vi "RT Image stream to FPGA.vi"() -> ()   [LabVIEW 2015]
uses:
  <vilib>/userdefined/High Color/IMAQdx.ctl
  <vilib>/vision/driver/IMAQdx.llb/IMAQdx Acquisition Mode.ctl
  <vilib>/vision/driver/IMAQdx.llb/IMAQdx Buffer Number Mode.ctl
  <vilib>/FPGAPlugInAG/cRIO-9030/niLvFpga_Open_cRIO-9030.vi
  <vilib>/rvi/interface/common/dynamic/niFpgaDynamicAddResources.vi
  <vilib>/FPGAPlugInAG/Dynamic/niLvFpga_Download_Dynamic.vi
  <vilib>/FPGAPlugInAG/Dynamic/niLvFpga_Run_Dynamic.vi
  <vilib>/visionFPGA/Basics/Configure Image Transfer to Target/IMAQ FPGA Configure Image Transfer to Target U8.vi
  <vilib>/visionFPGA/Basics/Configure Image Transfer from Target/IMAQ FPGA Configure Image Transfer from Target U8.vi
  <vilib>/visionFPGA/Basics/Image Transfer from Target/IMAQ FPGA Image Transfer from Target U8.vi
  <vilib>/FPGAPlugInAG/Dynamic/niLvFpga_Close_Dynamic.vi
  <vilib>/visionFPGA/Basics/Image Transfer to Target/IMAQ FPGA Image Transfer to Target U8.vi
  <vilib>/rvi/interface/nirviOpenFPGA/nirviOpenFPGA.xnode
  FPGA Bitfiles/BELKINEAGLE_FPGATarget_FPGAIPChainV1_CFyF0ro37YQ.lvbitx
  FPGA IP Chain V1.vi
  <vilib>/rvi/interface/nirviMethod/nirviMethod.xnode
  <vilib>/rvi/interface/nirviCloseFPGA/nirviCloseFPGA.xnode
  <vilib>/vision/driver/NI_Vision_Acquisition_Software.lvlib
  <resource>/objmgr/imaqdx.rc
  <vilib>/visionFPGA/NI_VDM_FPGA_Basics.lvlib
panel:
  in  "Camera":T1
  out "Error Out":errorcluster
  out "Image":T2(plugin-control)
  in  "Stop":bool
  # "Overview: Demonstrates how to acquire an image from a camera using the IMAQdx API, transfer the image to a FPGA target for processing, and retrieve the processed image for display or further processing on the host.\nRequirements:\n- LabVIEW FPGA\n- Vision Acquisition Software\n- Vision Development Module\nInstructions:\n1. Select a Camera\n2. Run the VI."
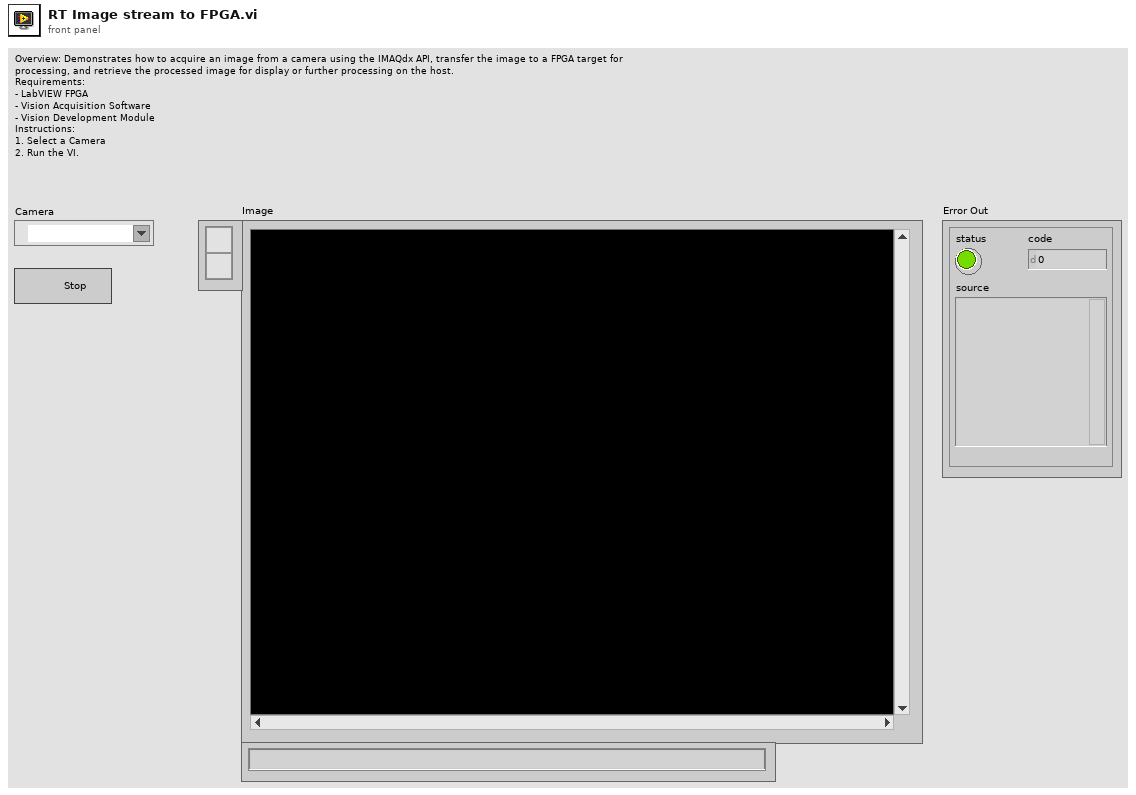
[diagram p1: front panel]
types:
  T1 = typedef "IMAQdx.ctl" = refnum<k21>
  T2 = typedef "IMAQ Image.ctl" = refnum<image>
  T3 = typedef "Image Type" = u32
  T4 = typedef "NI_Vision_Acquisition_Software.lvlib/IMAQdx Acquisition Mode.ctl" = enum32{"One Shot", "Continuous"}
  T5 = typedef "NI_Vision_Acquisition_Software.lvlib/IMAQdx Buffer Number Mode.ctl" = enum32{"Next", "Last", "Buffer Number", "Every", "Last New"}
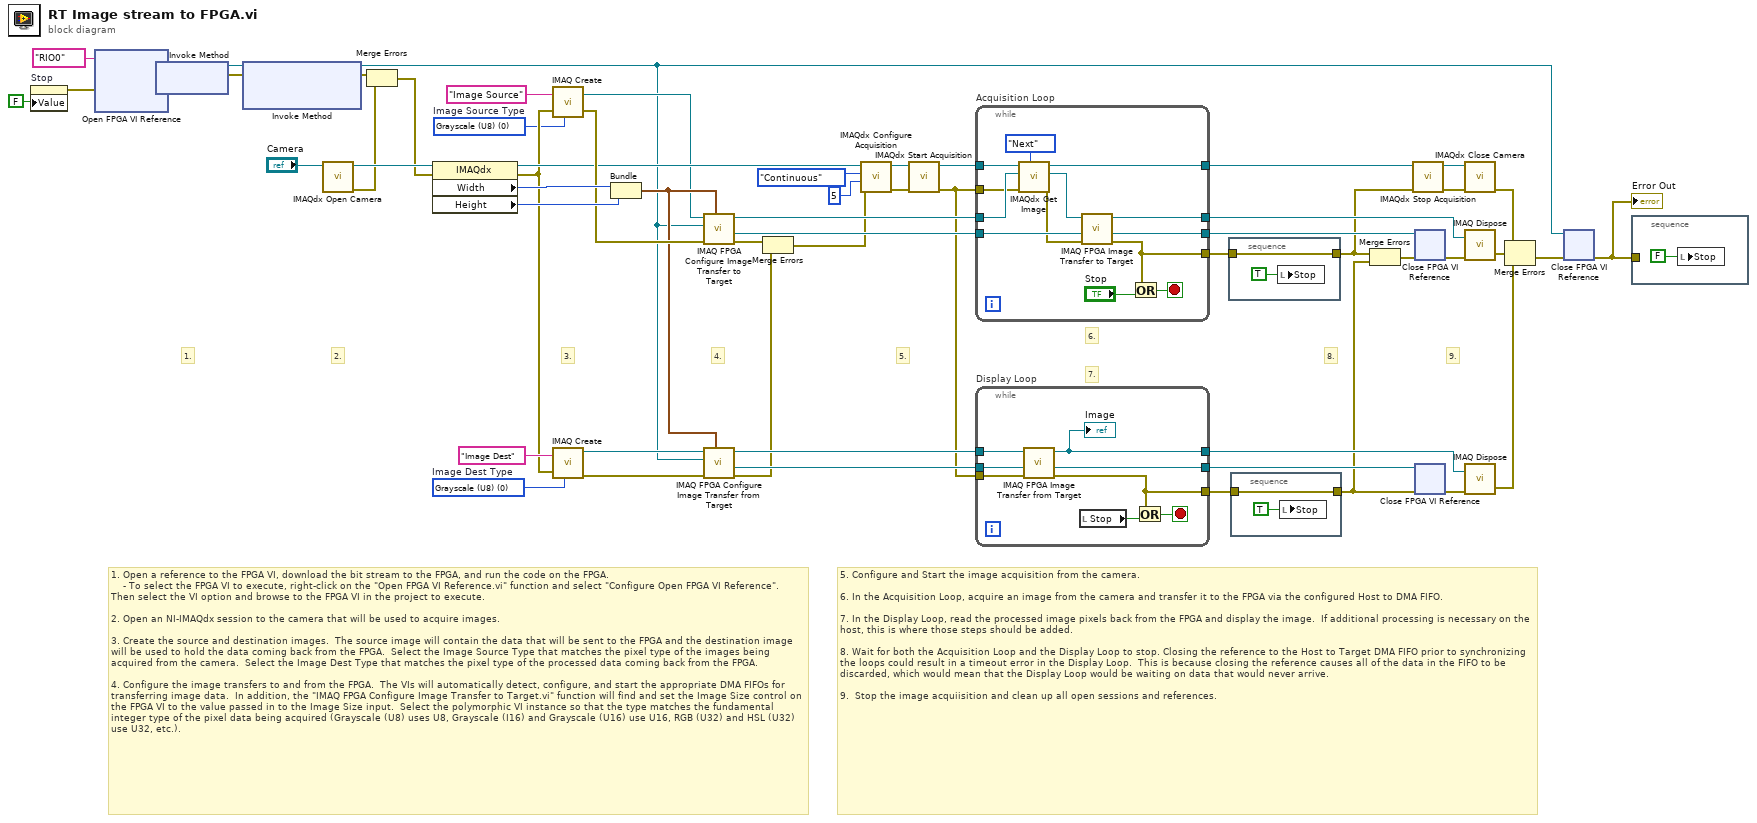
[diagram p0: block diagram]
diagram:
  w10 = T3 0 items=["Grayscale (U8)", "Grayscale (I16)", "Grayscale (SGL)", "Complex (CSG)", "RGB (U32)", "HSL (U32)", "RGB (U64)", "Grayscale (U16)"]  # Image Dest Type
  w11 = T3 0 items=["Grayscale (U8)", "Grayscale (I16)", "Grayscale (SGL)", "Complex (CSG)", "RGB (U32)", "HSL (U32)", "RGB (U64)", "Grayscale (U16)"]  # Image Source Type
  # "5. Configure and Start the image acquisition from the camera.\n\n6. In the Acquisition Loop, acquire an image from the camera and transfer it to the FPGA via the configured Host to DMA FIFO.\n\n7. In the Display Loop, read the processed image pixels back from the FPGA and display the image.  If additional processing is necessary on the host, this is where those steps should be added.\n\n8. Wait for both the Acquisition Loop and the Display Loop to stop. Closing the reference to the Host to Target DMA FIFO prior to synchronizing the loops could result in a timeout error in the Display Loop.  This is because closing the reference causes all of the data in the FIFO to be discarded, which would mean that the Display Loop would be waiting on data that would never arrive.\n\n9.  Stop the image acquiisition and clean up all open sessions and references."
  # "1. Open a reference to the FPGA VI, download the bit stream to the FPGA, and run the code on the FPGA.\n    - To select the FPGA VI to execute, right-click on the \"Open FPGA VI Reference.vi\" function and select \"Configure Open FPGA VI Reference\".  Then select the VI option and browse to the FPGA VI in the project to execute.\n\n2. Open an NI-IMAQdx session to the camera that will be used to acquire images.\n\n3. Create the source and destination images.  The source image will contain the data that will be sent to the FPGA and the destination image will be used to hold the data coming back from the FPGA.  Select the Image Source Type that matches the pixel type of the images being acquired from the camera.  Select the Image Dest Type that matches the pixel type of the processed data coming back from the FPGA.\n\n4. Configure the image transfers to and from the FPGA.  The VIs will automatically detect, configure, and start the appropriate DMA FIFOs for transferring image data.  In addition, the \"IMAQ FPGA Configure Image Transfer to Target.vi\" function will find and set the Image Size control on the FPGA VI to the value passed in to the Image Size input.  Select the polymorphic VI instance so that the type matches the fundamental integer type of the pixel data being acquired (Grayscale (U8) uses U8, Grayscale (I16) and Grayscale (U16) use U16, RGB (U32) and HSL (U32) use U32, etc.)."
  # "9."
  # "8."
  # "7."
  # "6."
  # "5."
  # "4."
  # "3."
  # "2."
  # "1."
  n1 = property on="Stop" class="Bool (strict)"("Value"=FALSE ("Stop")) -> (error out=w55:errorcluster)  [unwired: 2 in, 1 out]
  n2 = xnode "Open FPGA VI Reference"("error in"=w55, "resource name"=tag "RIO0") -> ("FPGA VI Reference Out"=w51:refnum<k20>, "error out"=w52:errorcluster)
  n3 = xnode "Invoke Method"("FPGA VI Reference In"=w51, "error in"=w52) -> ("FPGA VI Reference Out"=w54:refnum<k20>, "error out"=w53:errorcluster)
  n4 = xnode "Invoke Method"("FPGA VI Reference In"=w54, "error in"=w53) -> ("FPGA VI Reference Out"=w12:refnum<k20>, "error out"=w34:errorcluster)  [unwired: 1 in]
  n5 = call <vilib>:"IMAQdx Open Camera.vi"("Session In"="Camera") -> ("error out"=w19:errorcluster, "Session Out"=w20:T1)  [unwired: 9 in]
  n6 = Merge Errors(w34, w19) -> (w18:errorcluster)
  n7 = property class="IMAQdx"(reference=w20, error in=w18) -> (reference out=w27:T1, error out=w15:errorcluster, "Width"=w37:u32, "Height"=w36:u32)
  n8 = call "IMAQ Create"("Image Name"="Image Source", "Image Type"=w11, "error in (no error)"=w15) -> ("New Image"=w25:T2, "error out"=w33:errorcluster)  [unwired: 2 in]
  n9 = call "IMAQ Create"("Image Name"="Image Dest", "Image Type"=w10, "error in (no error)"=w15) -> ("New Image"=w14:T2, "error out"=w13:errorcluster)  [unwired: 2 in]
  n10 = Bundle("Width"=w37, "Height"=w36) -> (w32:cluster{"Width":u32, "Height":u32})  [unwired: 1 in]
  n11 = call-poly <vilib>:"IMAQ FPGA Configure Image Transfer to Target.vi"("Image Size"=w32, "error in (no error)"=w33, "FPGA VI Reference In"=w12, "Image"=w25) -> ("error out"=w4:errorcluster, "DMA FIFO Reference Out"=w49:refnum<k20>, "Image Out"=w50:T2)  [unwired: 4 in, 1 out]
  n12 = call-poly <vilib>:"IMAQ FPGA Configure Image Transfer from Target.vi"("Image Size"=w32, "error in (no error)"=w13, "FPGA VI Reference In"=w12, "Image"=w14) -> ("error out"=w2:errorcluster, "DMA FIFO Reference Out"=w47:refnum<k20>, "Image Out"=w48:T2)  [unwired: 5 in]
  n13 = Merge Errors(w4, w2) -> (w3:errorcluster)
  n14 = call <vilib>:"IMAQdx Configure Acquisition.vi"("error in"=w3, "Number of Buffers"=u32 5, "Continuous?"=IMAQdx_Acquisition_Mode."Continuous", "Session In"=w27) -> ("error out"=w30:errorcluster, "Session Out"=w31:T1)  [unwired: 6 in]
  n15 = call <vilib>:"IMAQdx Start Acquisition.vi"("error in"=w30, "Session In"=w31) -> ("error out"=w1:errorcluster, "Session Out"=w26:T1)  [unwired: 8 in]
  n16 = while "Acquisition Loop" {
    tunnel: [w59] -> w8
    tunnel: w50 -> [w64]
    tunnel: w49 -> [w69]
    tunnel: [w68] -> w9
    tunnel: [w67] -> w46
    tunnel: w26 -> [w65]
    tunnel: [w63] -> w22
    tunnel: w1 -> [w60]
    stop <- w70 stop-if-true
    n17 = call <vilib>:"IMAQdx Get Image.vi"("Buffer Number Mode (Next)"=IMAQdx_Buffer_Number_Mode."Next", "error in"=w60, "Image In"=w64, "Session In"=w65) -> ("error out"=w61:errorcluster, "Image Out"=w62:T2, "Session Out"=w63:T1)  [unwired: 4 in, 1 out]
    n18 = call-poly <vilib>:"IMAQ FPGA Image Transfer to Target.vi"("error in (no error)"=w61, "DMA FIFO Reference In"=w69, "Image"=w62) -> ("error out"=w59:errorcluster, "DMA FIFO Reference Out"=w68:refnum<k20>, "Image Out"=w67:T2)  [unwired: 6 in]
    n19 = Or(x=w59, y="Stop") -> (x .or. y?=w70:bool)
  }
  n20 = while "Display Loop" {
    tunnel: w48 -> [w78]
    tunnel: [w77] -> w43
    tunnel: w1 -> [w76]
    tunnel: w47 -> [w75]
    tunnel: [w74] -> w44
    tunnel: [w73] -> w41
    stop <- w79 stop-if-true
    n21 = call-poly <vilib>:"IMAQ FPGA Image Transfer from Target.vi"("error in (no error)"=w76, "DMA FIFO Reference In"=w75, "Image"=w78) -> ("error out"=w73:errorcluster, "DMA FIFO Reference Out"=w74:refnum<k20>, "Image Out"=w77:T2)  [unwired: 6 in]
    "Image" <- w77
    n22 = local read "Stop"() -> (w72:bool)
    n23 = Or(x=w73, y=w72) -> (x .or. y?=w79:bool)
  }
  n24 = stacked-sequence {
    tunnel: w8 -> [w80]
    tunnel: [w80] -> w5
    frame #0 {
      n25 = local write "Stop"(TRUE ("Stop")) -> ()
    }
  }
  n26 = stacked-sequence {
    tunnel: w41 -> [w82]
    tunnel: [w82] -> w7
    frame #0 {
      n27 = local write "Stop"(TRUE ("Stop")) -> ()
    }
  }
  n28 = Merge Errors(w5, w7) -> (w6:errorcluster)
  n29 = call <vilib>:"IMAQdx Stop Acquisition.vi"("error in"=w5, "Session In"=w22) -> ("error out"=w23:errorcluster, "Session Out"=w24:T1)  [unwired: 8 in]
  n30 = xnode "Close FPGA VI Reference"("FPGA VI Reference In"=w9, "error in"=w6) -> ("error out"=w45:errorcluster)
  n31 = xnode "Close FPGA VI Reference"("FPGA VI Reference In"=w44, "error in"=w7) -> ("error out"=w42:errorcluster)
  n32 = call <vilib>:"IMAQdx Close Camera.vi"("error in"=w23, "Session In"=w24) -> ("error out"=w21:errorcluster)  [unwired: 9 in]
  n33 = call "IMAQ Dispose"("Image"=w46, "error in (no error)"=w45) -> ("error out"=w39:errorcluster)  [unwired: 4 in]
  n34 = call "IMAQ Dispose"("Image"=w43, "error in (no error)"=w42) -> ("error out"=w40:errorcluster)  [unwired: 4 in]
  n35 = Merge Errors(w21, w39, w40) -> (w17:errorcluster)
  n36 = xnode "Close FPGA VI Reference"("FPGA VI Reference In"=w12, "error in"=w17) -> ("error out"=w16:errorcluster)
  "Error Out" <- w16
  n37 = stacked-sequence {
    tunnel: w16 -> [_]
    frame #0 {
      n38 = local write "Stop"(FALSE ("Stop")) -> ()
    }
  }
